vi "calc_pixelhits_smeary.vi"(8 "error in":errorcluster, 10 "Lookup arrays":T1, 11 "Pixelhits array in":refnum<data-value>) -> (0 "error out":errorcluster, 3 "Pixelhits array out":refnum<data-value>)   [LabVIEW 2011, in "Fiberscope_library.lvlib"]
uses:
  Fiberscope_library.lvlib
  typedefs/lookup_arrays_ref_cluster.ctl
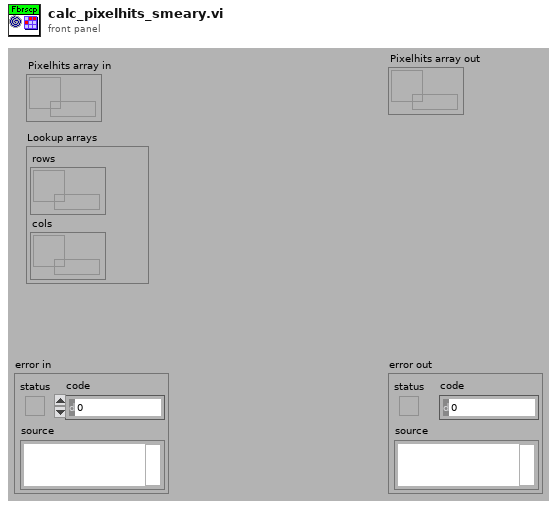
[diagram p1: front panel]
types:
  T1 = typedef "Fiberscope_library.lvlib/lookup_arrays_ref_cluster.ctl" = cluster{"rows":refnum<data-value>, "cols":refnum<data-value>}
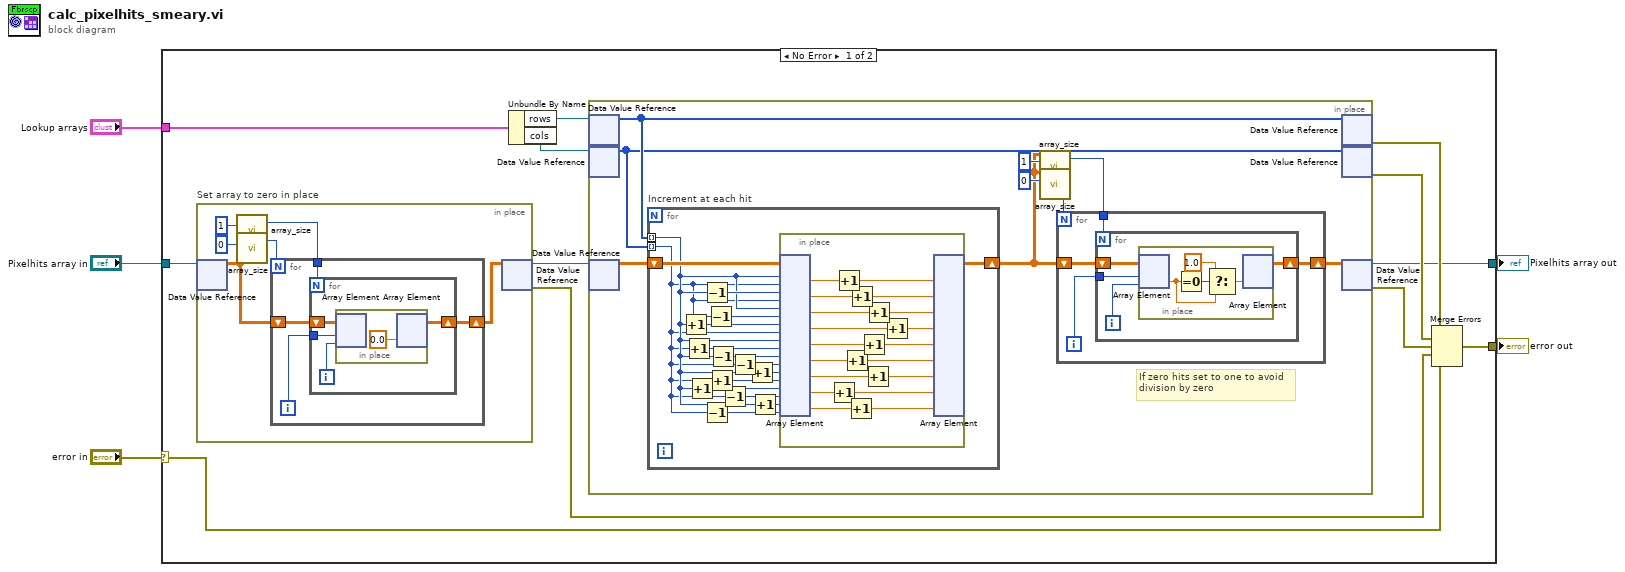
[diagram p0: block diagram]
diagram:
  n1 = case shown="No Error" "error in" {
    selector: "error in" -> [w6 w89]
    tunnel: [w9 w89] -> w4
    tunnel: [w8 w88] -> w2
    tunnel: "Pixelhits array in" -> [w7 w88]
    tunnel: "Lookup arrays" -> [w17 _]
    frame No Error {
      n2 = in-place "Set array to zero in place" {
        n3 = in-place-dvr #1(w7) -> (w20:dbl[][])  [unwired: 1 out]
        n4 = call "array_size.vi"("Array"=w20, "Dimension"=1) -> ("Dimension size"=w18:i32)  [unwired: 4 in]
        n5 = call "array_size.vi"("Array"=w20, "Dimension"=0) -> ("Dimension size"=w21:i32)  [unwired: 4 in]
        n6 = for {
          N: w21 -> [_]
          shift-right: [w25] -> w23
          shift-left: w20 -> [w27]
          tunnel: w18 -> [w24]
          i -> [w26]
          n7 = for {
            N: w24 -> [_]
            shift-right: [w28] -> w25
            shift-left: w27 -> [w31]
            tunnel: w26 -> [w30]
            i -> [w29]
            n8 = in-place {
              n9 = in-place-array #2(w31, w30, w29) -> ()  [unwired: 1 out]
              n10 = in-place-array #2(0.0 ("element")) -> (w28:dbl[][])  [unwired: 2 out]
            }
          }
        }
        n11 = in-place-dvr #1(w23) -> (w14:refnum<data-value>, w10:errorcluster)
      }
      n12 = Unbundle By Name(w17) -> ("rows"=w16:refnum<data-value>, "cols"=w15:refnum<data-value>)
      n13 = in-place {
        # "If zero hits set to one to avoid\ndivision by zero"
        n14 = in-place-dvr #3(w16) -> (w40:i32[])  [unwired: 1 out]
        n15 = in-place-dvr #4(w15) -> (w39:i32[])  [unwired: 1 out]
        n16 = in-place-dvr #5(w14) -> (w41:dbl[][])  [unwired: 1 out]
        n17 = for "Increment at each hit" {
          shift-right: [w68] -> w35
          shift-left: w41 -> [w69]
          tunnel: w39 -> [w54] mode=indexing
          tunnel: w40 -> [w56] mode=indexing
          n18 = Increment(x=w56) -> (x+1=w65:i32)
          n19 = Increment(x=w54) -> (x+1=w64:i32)
          n20 = Increment(x=w56) -> (x+1=w59:i32)
          n21 = Decrement(x=w56) -> (x-1=w67:i32)
          n22 = Decrement(x=w54) -> (x-1=w55:i32)
          n23 = Decrement(x=w54) -> (x-1=w66:i32)
          n24 = Increment(x=w54) -> (x+1=w60:i32)
          n25 = Decrement(x=w56) -> (x-1=w63:i32)
          n26 = Decrement(x=w54) -> (x-1=w57:i32)
          n27 = Decrement(x=w54) -> (x-1=w62:i32)
          n28 = Increment(x=w56) -> (x+1=w61:i32)
          n29 = Increment(x=w56) -> (x+1=w58:i32)
          n30 = in-place {
            n31 = in-place-array #6(w69, w56, w54, w67, w54, w56, w66, w65, w54, w56, w64, w63, w62, w61, w60, w59, w57, w58, w55) -> (w87:dbl, w85:dbl, w83:dbl, w81:dbl, w79:dbl, w77:dbl, w75:dbl, w74:dbl, w71:dbl)
            n32 = Increment(x=w74) -> (x+1=w72:dbl)
            n33 = Increment(x=w87) -> (x+1=w86:dbl)
            n34 = Increment(x=w77) -> (x+1=w76:dbl)
            n35 = Increment(x=w71) -> (x+1=w70:dbl)
            n36 = Increment(x=w85) -> (x+1=w84:dbl)
            n37 = Increment(x=w79) -> (x+1=w78:dbl)
            n38 = Increment(x=w75) -> (x+1=w73:dbl)
            n39 = Increment(x=w83) -> (x+1=w82:dbl)
            n40 = Increment(x=w81) -> (x+1=w80:dbl)
            n41 = in-place-array #6(w86, w84, w82, w80, w78, w76, w73, w72, w70) -> (w68:dbl[][])  [unwired: 18 out]
          }
        }
        n42 = call "array_size.vi"("Array"=w35, "Dimension"=1) -> ("Dimension size"=w34:i32)  [unwired: 4 in]
        n43 = call "array_size.vi"("Array"=w35, "Dimension"=0) -> ("Dimension size"=w33:i32)  [unwired: 4 in]
        n44 = for {
          N: w33 -> [_]
          shift-right: [w43] -> w38
          shift-left: w35 -> [w45]
          tunnel: w34 -> [w42]
          i -> [w44]
          n45 = for {
            N: w42 -> [_]
            shift-right: [w46] -> w43
            shift-left: w45 -> [w49]
            tunnel: w44 -> [w48]
            i -> [w47]
            n46 = in-place {
              n47 = in-place-array #7(w49, w48, w47) -> (w52:dbl)
              n48 = Equal To 0?(x=w52) -> (x = 0?=w53:bool)
              n49 = Select(t=1.0, s=w53, f=w52) -> (s? t:f=w50:dbl)
              n50 = in-place-array #7(w50) -> (w46:dbl[][])  [unwired: 2 out]
            }
          }
        }
        n51 = in-place-dvr #3(w40) -> (w13:errorcluster)  [unwired: 1 out]
        n52 = in-place-dvr #4(w39) -> (w12:errorcluster)  [unwired: 1 out]
        n53 = in-place-dvr #5(w38) -> (w8:refnum<data-value>, w11:errorcluster)
      }
      n54 = Merge Errors(w13, w12, w11, w10, w6) -> (w9:errorcluster)
    }
    frame Error {
    }
  }
  "error out" <- w4
  "Pixelhits array out" <- w2
